vi "HMT Launcher.vi"   [LabVIEW 2023]
uses:
  Hotel Management Tool Model/Hotel Management Tool Model/Hotel Management Tool Model.lvclass
  <vilib>/ActorFramework/Actor/Actor.lvclass
panel:
  # "Launch Hotel Management Tool"
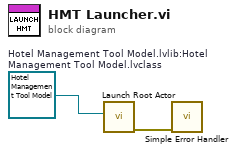
[diagram p0: block diagram]
diagram:
  w1 = refnum<class "Hotel Management Tool Model.lvclass"> refnum  # Hotel Management Tool Model.lvlib:Hotel Management Tool Model.lvclass
  n1 = call <vilib>:"Launch Root Actor.vi"("Actor"=w1) -> ("error out"=w2:errorcluster)  [unwired: 9 in, 1 out]
  n2 = call <vilib>:"Simple Error Handler.vi"("error in (no error)"=w2) -> ()  [unwired: 4 in, 5 out]
